vi "EventTCP.vi"() -> ()   [LabVIEW 2014]
panel:
  out "Connected":bool
  out "String":string
  out "Unique String":bool
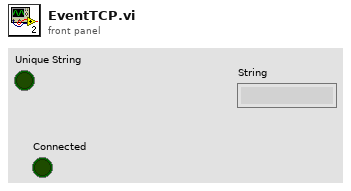
[diagram p1: front panel]
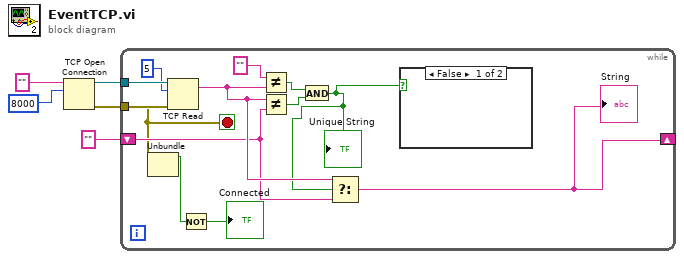
[diagram p0: block diagram]
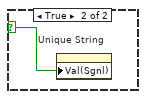
[diagram p2: hidden frame]
diagram:
  n1 = TCP Open Connection(address="", remote port or service name=8000) -> (connection ID=w3:refnum<k5>, error out=w2:errorcluster)  [unwired: 3 in]
  n2 = while {
    tunnel: w3 -> [w18]
    tunnel: w2 -> [w17]
    shift-right: [w9] -> _
    shift-left: "" -> [w11]
    stop <- w8 stop-if-true
    n3 = TCP Read(connection ID=w18, bytes to read=5, error in (no error)=w17) -> (data out=w12:string, error out=w8:errorcluster)  [unwired: 2 in, 1 out]
    n4 = Unbundle(w8) -> ("status"=w6:bool)  [unwired: 2 out]
    n5 = Not(x=w6) -> (.not. x?=→"Connected":bool)
    n6 = Not Equal?(x="", y=w12) -> (x != y?=w13:bool)
    n7 = Not Equal?(x=w12, y=w11) -> (x != y?=w14:bool)
    n8 = And(x=w13, y=w14) -> (x .and. y?=w10:bool)
    "Unique String" <- w10
    n9 = Select(t=w12, s=w10, f=w11) -> (s? t:f=w9:string)
    "String" <- w9
    n10 = case shown="False" w10 {
      selector: w10 -> [_ w19]
      frame False {
      }
      frame True {
        n11 = property on="Unique String" class="Bool (strict)"("Val(Sgnl)"=w19) -> ()  [unwired: 2 in, 2 out]
      }
    }
  }
